vi "OE2052_RS232_Query Data.vi"(0 "VISA resource name":refnum<visa-resource-name>, 11 "Error in (no error)":errorcluster caption="error out（no error）") -> (4 "VISA resource  out":refnum<visa-resource-name>, 6 "Data Array":dbl[](array[numeric]), 8 "Parameter Values":T1, 10 "Output String":string, 15 "Error out":errorcluster caption="error out")   [LabVIEW 2011]
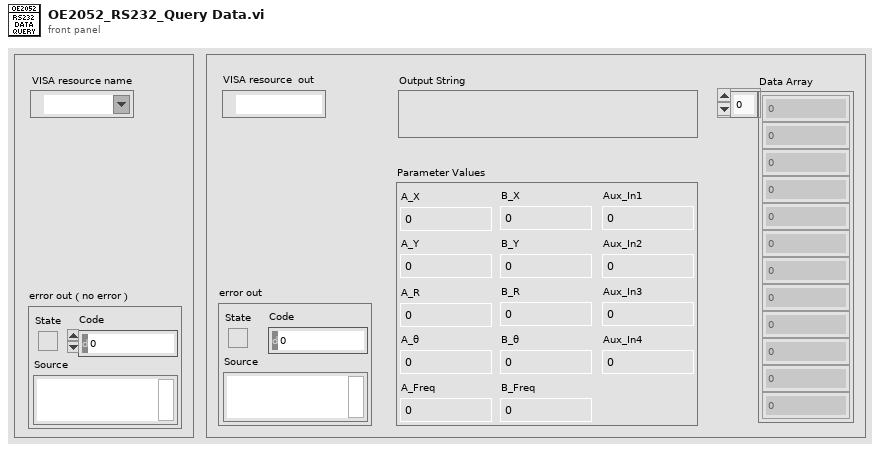
[diagram p1: front panel]
types:
  T1 = cluster{"A_X":dbl, "A_Y":dbl, "A_R":dbl, "A_θ":dbl, "A_Freq":dbl, "B_X":dbl, "B_Y":dbl, "B_R":dbl, "B_θ":dbl, "B_Freq":dbl, "Aux_In1":dbl, "Aux_In2":dbl, "Aux_In3":dbl, "Aux_In4":dbl}
  T2 = cluster{dbl, dbl, dbl, dbl, dbl, dbl, dbl, dbl, dbl, dbl, dbl, dbl, dbl, dbl}
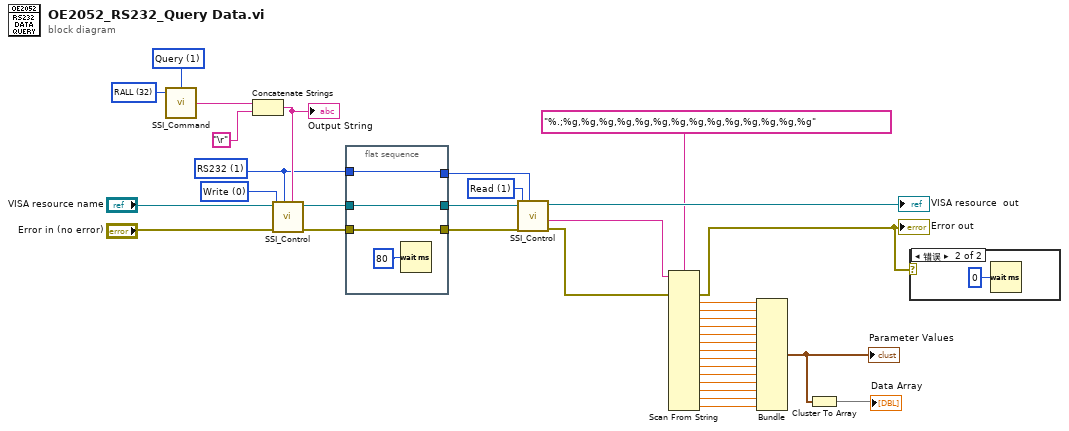
[diagram p0: block diagram]
diagram:
  w6 = u16 1 items=["USB"=0, "RS232"=1, "Ethernet"=3] ("Remote Mode")
  w8 = u16 32 items=["ISRC", "IGND", "ICPL", "ILIN", "PHAS", "FMOD", "RSLP", "FREQ", "SWPT", "SLLM", "SULM", "SSLL", "SSLG", "STLM", "SWRM", "IRNG", "SENS", "RMOD", "OFLT", "OFSL", "SYNC", "DMOD", "HARM", "DARB", "SWVT", "SLVL", "SVLL", "SVUL", "SVSL", "SVSG", "SVTM", "SVRM", "RALL", "SNAP", "OUTP", "OAUX", "COUT", "CAUX", "COFP", "CEXP", "FPOP", "OEXP", "*IDN", "*RST", "OVLD", "INOV", "GNOV", "*PLL", "SSET", "RSET", "AGAN", "APHS", "ARSV", "ASCL", "EQCD", "EQCS", "SPED", "SRAT", "SLEN", "SSLE", "STRG", "SPRM", "STRD", "PAUS", "RSET", "SPTS", "TRCA", "TEMP", "RSTU", "INHZ", "DEQU", "SADD", "ARNG", "CSPE", "ISRCD", "IGNDD", "ICPLD", "ILIND", "PHASD", "FMODD", "RSLPD", "FREQD", "SWPTD", "SLLMD", "SULMD", "SSLLD", "SSLGD", "STLMD", "SWRMD", "SENSD", "RMODD", "OFLTD", "OFSLD", "SYNCD", "HARMD", "EQCDD", "EQCSD", "SNAPD", "OUTPD", "SWVTD", "SLVLD", "SVLLD", "SVULD", "SVSLD", "SVSGD", "SVTMD", "SVRMD", "SVDCD", "ARSVD", "AGAND", "APHSD", "ASCLD", "FPOPD", "CAUXD", "OEXPD", "SPEDD", "SRATD", "SLEND", "SSLED", "STRGD", "SPRMD", "STRDD", "PAUSD", "RESTD", "SPTSD", "TRCAD", "*IDND", "*RSTD", "INOVD", "GNOVD", "*PLLD", "SSETD", "RSETD", "RALLD"] ("Command Type")
  w4 = u16 1 items=["Set", "Query"] ("Opera")
  w28 = u16 1 items=["Write", "Read"] ("Control")
  w33 = u16 0 items=["Write", "Read"] ("Control")
  n1 = call "SSI_Command.vi"("Opera"=w4, "Command Type"=w8) -> ("Output string"=w7:string)  [unwired: 2 in]
  n2 = Concatenate Strings(w7, "\r") -> (w9:string)
  "Output String" <- w9
  n3 = call "SSI_Control.vi"("Write Buffer"=w9, "Remote Mode"=w6, "Error in (no error)"="Error in (no error)", "Control"=w33, "VISA resource name"="VISA resource name") -> ("Error out"=w31:errorcluster, "VISA resource  out"=w32:refnum<visa-resource-name>)  [unwired: 3 in, 2 out]
  n4 = flat-sequence {
    tunnel: w32 -> [w40]
    tunnel: w31 -> [w39]
    tunnel: [w40] -> w30
    tunnel: [w39] -> w29
    tunnel: [w37] -> w27
    tunnel: w6 -> [w37]
    frame #0 {
      n5 = Wait (ms)(milliseconds to wait=u32 80 ("等待时间（毫秒）")) -> ()  [unwired: 1 out]
    }
  }
  n6 = call "SSI_Control.vi"("Remote Mode"=w27, "Error in (no error)"=w29, "Control"=w28, "VISA resource name"=w30) -> ("Error out"=w26:errorcluster, "Read Buffer"=w5:string, "VISA resource  out"=→"VISA resource  out":refnum<visa-resource-name>)  [unwired: 4 in, 1 out]
  n7 = Scan From String(format string="%.;%g,%g,%g,%g,%g,%g,%g,%g,%g,%g,%g,%g,%g,%g" ("格式字符串"), input string=w5, error in=w26) -> (error out=w1:errorcluster, output 1=w25:dbl, output 2=w24:dbl, output 3=w23:dbl, output 4=w22:dbl, output 5=w21:dbl, output 6=w19:dbl, output 7=w18:dbl, output 8=w17:dbl, output 9=w16:dbl, output 10=w15:dbl, output 11=w14:dbl, output 12=w13:dbl, output 13=w12:dbl, output 14=w11:dbl)  [unwired: 15 in, 2 out]
  "Error out" <- w1
  n8 = Bundle(w25, w24, w23, w22, w21, w19, w18, w17, w16, w15, w14, w13, w12, w11) -> (w2:T2)  [unwired: 1 in]
  "Parameter Values" <- w2
  n9 = Cluster To Array(cluster=w2) -> (array=→"Data Array":dbl[])
  n10 = case shown="错误" w1 {
    frame No Error {
    }
    frame Error {
      n11 = Wait (ms)(milliseconds to wait=u32 0 ("等待时间（毫秒）")) -> ()  [unwired: 1 out]
    }
  }
